vi "createCommandString.vi"(8 "error in (no error)":errorcluster, 11 "TEI9150 in":refnum<class "TEI9150.lvclass">) -> (0 "error out":errorcluster, 3 "TEI9150 out":refnum<class "TEI9150.lvclass">)   [LabVIEW 2015, in "TEI9150.lvclass"]
uses:
  TEI9150.lvclass
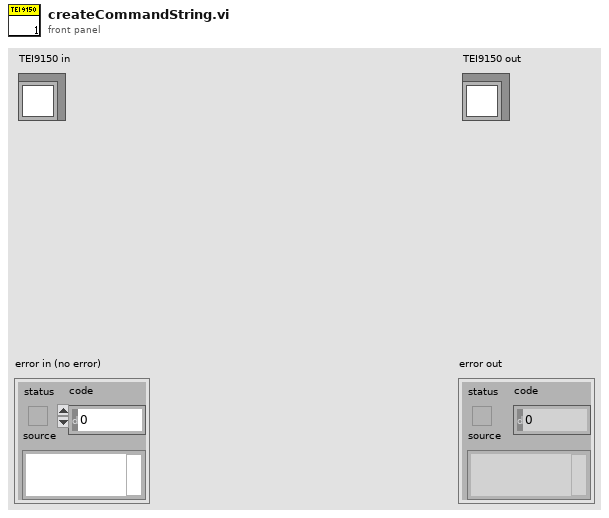
[diagram p1: front panel]
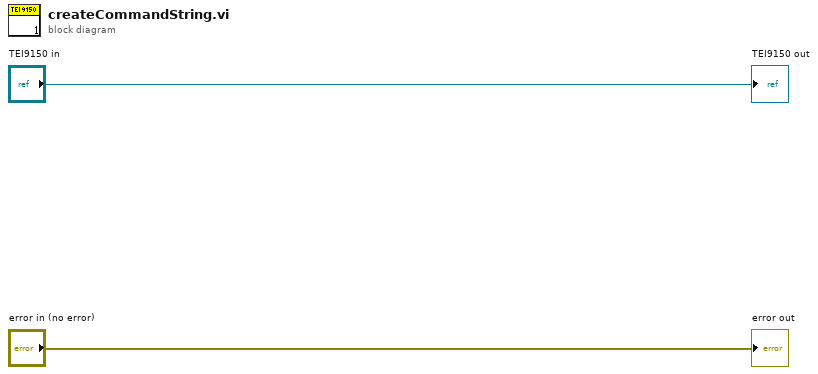
[diagram p0: block diagram]
diagram:
  "error out" <- "error in (no error)"
  "TEI9150 out" <- "TEI9150 in"
